vi "GetDevicesByMetadataObj.vi"(8 "error in (no error)":errorcluster, 11 "MetaDataObj in":refnum<class "MetaDataObj.lvclass">) -> (0 "error out":errorcluster, 1 "Found?":bool, 2 "Supported Devices":u32[](array[numeric]), 3 "MetaDataObj Out":refnum<class "MetaDataObj.lvclass">)   [LabVIEW 2021, in "myRIOMetaDataObj.lvclass"]
uses:
  myRIOMetaDataObj.lvclass
  <resource>/dialog/NewProjectWizard/MetaDataObj/MetaDataObj.lvclass
  <resource>/dialog/NewProjectWizard/MetaDataObj/Accessors/Read Title.vi
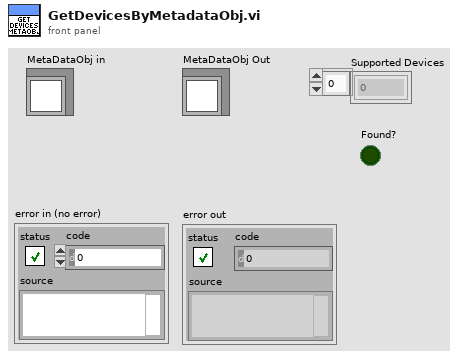
[diagram p1: front panel]
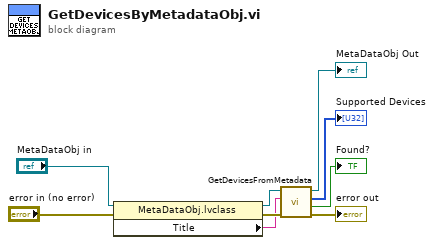
[diagram p0: block diagram]
diagram:
  n1 = property class="MetaDataObj.lvclass"(reference="MetaDataObj in", error in="error in (no error)") -> (reference out=w4:refnum<class "MetaDataObj.lvclass">, error out=w6:errorcluster, "Title"=w5:string)
  n2 = call "GetDevicesFromMetadata.vi"("error in (no error)"=w6, "Title"=w5, "MetaDataObj in"=w4) -> ("error out"=→"error out":errorcluster, "Found?"=→"Found?":bool, "Supported Devices"=→"Supported Devices":u32[], "MetaDataObj Out"=→"MetaDataObj Out":refnum<class "MetaDataObj.lvclass">)  [unwired: 5 in]
